vi "Michelle Fahrenheit-Celcius (10-16).vi"() -> ()   [LabVIEW 2012]
panel:
  out "Celcius":dbl
  in  "Fahrenheit":dbl
  in  "Celcius":bool
  in  "Celcius":dbl
  out "Fahrenheit":dbl
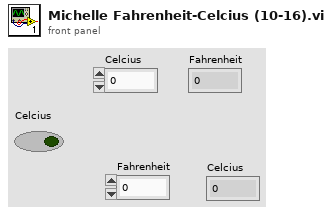
[diagram p1: front panel]
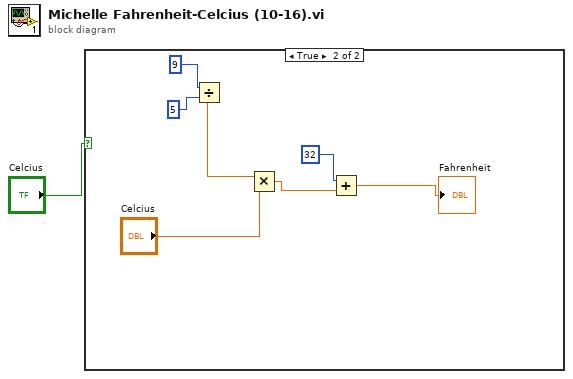
[diagram p0: block diagram]
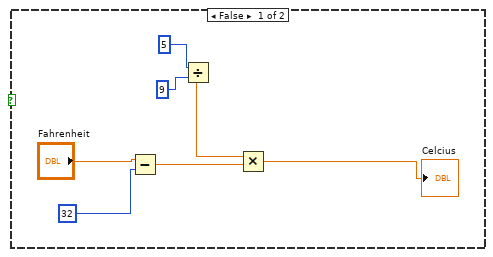
[diagram p2: hidden frame]
diagram:
  n1 = case shown="True" "Celcius" {
    frame False {
      n2 = Subtract(x="Fahrenheit", y=32) -> (x-y=w3:dbl)
      n3 = Divide(x=5, y=9) -> (x/y=w6:dbl)
      n4 = Multiply(x=w6, y=w3) -> (x*y=→"Celcius":dbl)
    }
    frame True {
      n5 = Divide(x=9, y=5) -> (x/y=w12:dbl)
      n6 = Multiply(x=w12, y="Celcius") -> (x*y=w13:dbl)
      n7 = Add(x=32, y=w13) -> (x+y=→"Fahrenheit":dbl)
    }
  }
